vi "XY Dialog - Initialize Tree.vi"(8 "error in (no error)":errorcluster, 10 "TreeAliasBrowserWF":refnum<k24>(container), 11 "GraphData.System.Root":refnum<k24>) -> (0 "error out":errorcluster, 3 "Event Registration Refnum":refnum<event-registration>)   [LabVIEW 2020, in "Workspace MultiY Graph.lvlib"]
uses:
  Workspace MultiY Graph.lvlib
  NationalInstruments.VeriStand.SystemStorage
  NationalInstruments.VeriStand.SystemStorageUI
  <vilib>/NI VeriStand/UI Controls/Tree and Alias Browser/Net Event Data Ref.ctl
  <vilib>/NI VeriStand/UI Controls/Tree and Alias Browser/Net Event Data.ctl
  <vilib>/NI VeriStand/UI Controls/Tree and Alias Browser/Net Event.ctl
  <vilib>/NI VeriStand/UI Controls/Tree and Alias Browser/NI_VS UI Tree Alias Browser.lvlib
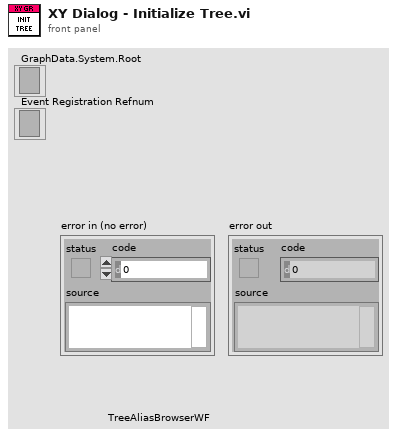
[diagram p1: front panel]
types:
  T1 = typedef "NI_VS UI Tree Alias Browser.lvlib/Callback Type.ctl" = cluster{"Net Callbacks":refnum<k27>[], "Event":T2}
  T2 = typedef "NI_VS UI Tree Alias Browser.lvlib/Net Event Data Ref.ctl" = refnum<user-event>
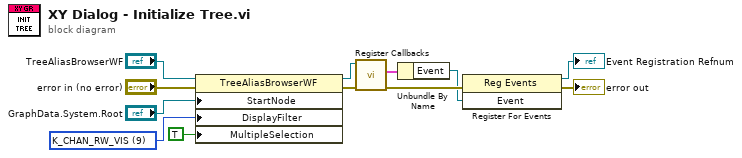
[diagram p0: block diagram]
diagram:
  w9 = u8 9 items=["K_CHAN_R", "K_CHAN_W", "K_CHAN_RW", "K_CHAN_VOLT", "K_CHAN_FAULT", "K_ALL", "K_CUSTOM", "K_CHAN_R_VIS", "K_CHAN_W_VIS", "K_CHAN_RW_VIS", "K_CHAN_VOLT_VIS", "K_CHAN_FAULT_VIS", "K_WAVE", "K_WAVE_VIS", "K_WAVE_DBL", "K_WAVE_CDB", "K_WAVE_DBL_VIS", "K_WAVE_CDB_VIS"] ("DisplayFilter")
  n1 = property class="TreeAliasBrowserWF"(reference="TreeAliasBrowserWF", error in="error in (no error)", "StartNode"="GraphData.System.Root", "DisplayFilter"=w9, "MultipleSelection"=TRUE) -> (reference out=w7:refnum<k24>, error out=w6:errorcluster)
  n2 = call <vilib>:"Register Callbacks.vi"("error in (no error)"=w6, "Tree Alias"=w7) -> ("error out"=w4:errorcluster, "Callbacks"=w5:T1)  [unwired: 7 in, 1 out]
  n3 = Unbundle By Name(w5) -> ("Event"=w3:T2)
  n4 = register-events(error in=w4, w3) -> (reference out=→"Event Registration Refnum":refnum<event-registration>, error out=→"error out":errorcluster)  [unwired: 1 in]
